vi "Read Transmission Spectrum.vi"(0 "VISA IN":refnum<visa-resource-name>="COM1" caption="serial number", 5 "error in (no error)":errorcluster caption="错误输入（无错误）") -> (14 "VISA OUT":refnum<visa-resource-name>, 15 "DATA":u8[](array[numeric]) format="%02x", 19 "error out":errorcluster caption="错误输出")   [LabVIEW 2013]
uses:
  <vilib>/Utility/file.llb/Write To Spreadsheet File (I64).vi
panel:
  out "Numeric":i32
  out "File path":path
  in  "Times":i32=10
  in  "STOP":bool
  out "XY Graph":cluster{i32[], u32[]}(graph)
  out "read buffer":string
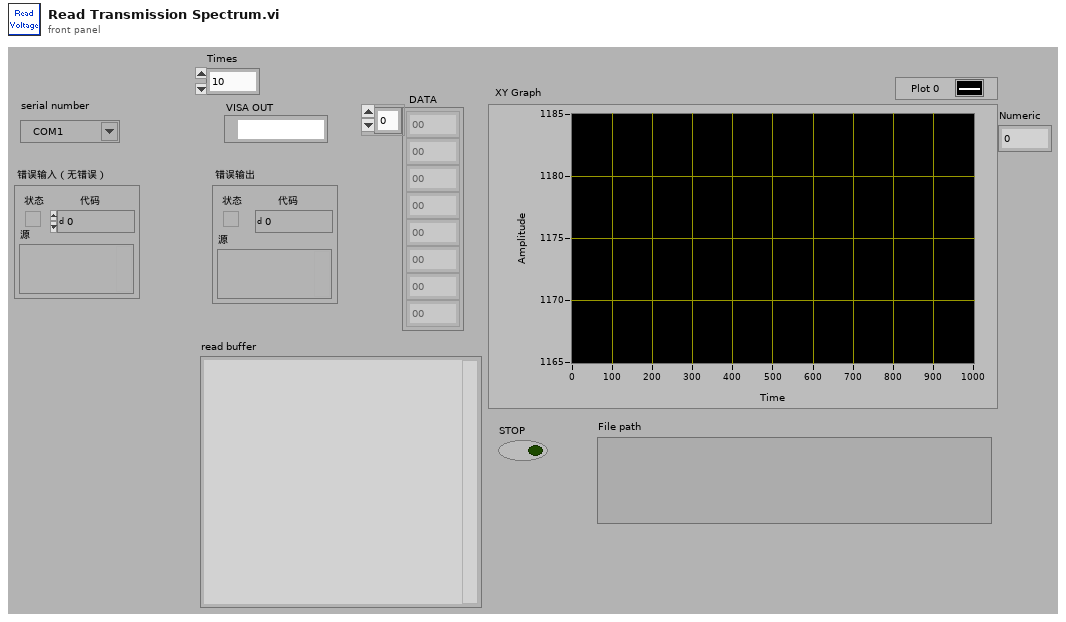
[diagram p1: front panel]
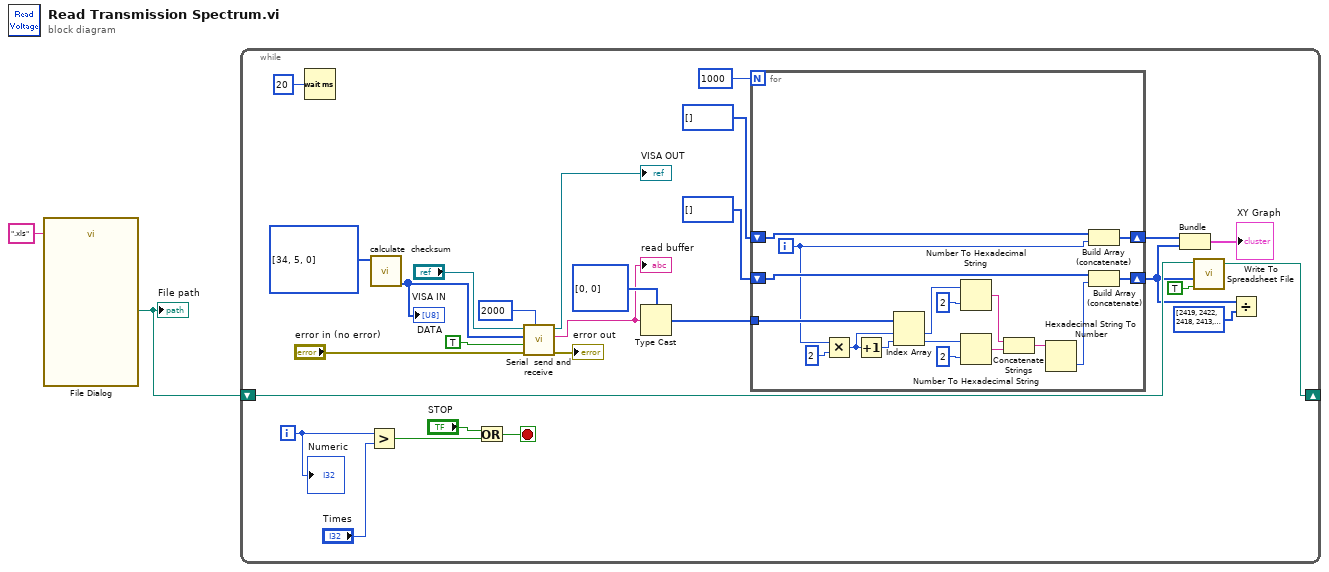
[diagram p0: block diagram]
diagram:
  n1 = call "File Dialog"("default name"=".xls") -> ("selected path"=w1:path)  [unwired: 11 in, 3 out]
  "File path" <- w1
  n2 = while {
    shift-right: [w6] -> _
    shift-left: w1 -> [w5]
    i -> [w10]
    stop <- w13 stop-if-true
    n3 = Wait (ms)(milliseconds to wait=u32 20) -> ()  [unwired: 1 out]
    n4 = Greater?(x=w10, y="Times") -> (0:w11:bool)
    n5 = call "calculate  checksum.vi"("front command"=u8[] [34, 5, 0]) -> ("DATA"=w29:u8[])  [unwired: 9 in, 1 out]
    "DATA" <- w29
    n6 = Or(x="STOP", y=w11) -> (x .or. y?=w13:bool)
    n7 = call "Serial  send and receive.vi"("读取字节总数"=u32 2000, "error in (no error)"="error in (no error)", "读取"=TRUE, "command"=w29, "VISA IN"="VISA IN") -> ("error out"=→"error out":errorcluster, "read buffer"=w14:string, "VISA OUT"=→"VISA OUT":refnum<visa-resource-name>)  [unwired: 2 in, 2 out]
    "read buffer" <- w14
    n8 = Type Cast(type=u8[] [0, 0], x=w14) -> (*(type *) &x=w20:u8[])
    n9 = for {
      N: 1000 -> [_]
      tunnel: w20 -> [w44]
      shift-right: [w35] -> w3
      shift-left: u32[] [] -> [w33]
      shift-right: [w31] -> w16
      shift-left: i32[] [] -> [w30]
      i -> [w32]
      n10 = Multiply(x=w32, y=i16 2 ("宽度(-)")) -> (x*y=w37:i32)
      n11 = Increment(x=w37) -> (x+1=w36:i32)
      n12 = Index Array(array=w44, index #1=w37, index #2=w36) -> (element #1=w46:u8, element #2=w43:u8)
      n13 = Number To Hexadecimal String(1:i16 2 ("宽度(-)"), 2:w46) -> (0:w45:string)
      n14 = Number To Hexadecimal String(1:i16 2 ("宽度(-)"), 2:w43) -> (0:w42:string)
      n15 = Concatenate Strings(w45, w42) -> (w39:string)
      n16 = Hexadecimal String To Number(string=w39) -> (number=w34:u32)  [unwired: 2 in, 1 out]
      n17 = Build Array (concatenate)(w30, w32) -> (w31:i32[])
      n18 = Build Array (concatenate)(w33, w34) -> (w35:u32[])
    }
    n19 = Bundle(w16, w3) -> (→"XY Graph":cluster{i32[], u32[]})  [unwired: 1 in]
    n20 = call-poly <vilib>:"Write To Spreadsheet File.vi"("append to file? (new file:F)"=TRUE, "1D data"=w3, "file path (dialog if empty)"=w5) -> ("new file path (Not A Path if cancelled)"=w6:path)  [unwired: 5 in]
    n21 = Divide(x=w3, y=u32[] [2419, 2422, 2418, 2413, 2407, 2401, 2394, 2390, 2384, 2380, 2372, 2366, 2351, 2347, 2343, 2338, 2334, 2327, 2321, 2317, 2316, 2311, 2305, 2301, 2294, 2289, 2285, 2281, 2276, 2272, 2268, 2266, 2260, 2255, 2253, 2249, 2246, 2243, 2237, 2233, 2231, 2226, 2222, 2218, 2216, 2213, 2207, 2206, 2203, 2198, 2196, 2192, 2191, 2187, 2185, 2182, 2176, 2177, 2175, 2175, 2170, 2166, 2161, 2160, 2155, 2152, 2149, 2149, 2146, 2142, 2141, 2139, 2137, 2135, 2134, 2131, 2127, 2125, 2124, 2122, 2120, 2118, 2116, 2114, 2110, 2110, 2109, 2108, 2105, 2102, 2104, 2098, 2101, 2097, 2094, 2093, 2098, 2093, 2093, 2092, 2087, 2085, 2083, 2082, 2082, 2081, 2080, 2079, 2077, 2076, 2074, 2073, 2073, 2071, 2060, 2069, 2069, 2068, 2069, 2066, 2065, 2065, 2065, 2063, 2063, 2061, 2058, 2060, 2058, 2057, 2056, 2056, 2059, 2056, 2059, 2056, 2058, 2057, 2052, 2052, 2052, 2053, 2052, 2052, 2052, 2051, 2051, 2049, 2051, 2050, 2048, 2050, 2051, 2049, 2049, 2049, 2047, 2048, 2048, 2048, 2048, 2047, 2047, 2048, 2047, 2047, 2049, 2047, 2047, 2048, 2046, 2048, 2048, 2049, 2050, 2050, 2050, 2046, 2047, 2047, 2045, 2048, 2035, 2047, 2044, 2048, 2048, 2049, 2048, 2048, 2049, 2048, 2048, 2048, 2048, 2049, 2050, 2049, 2049, 2048, 2048, 2049, 2049, 2048, 2052, 2050, 2050, 2049, 2049, 2051, 2052, 2056, 2055, 2056, 2056, 2053, 2054, 2053, 2055, 2054, 2054, 2055, 2055, 2056, 2052, 2057, 2056, 2056, 2059, 2058, 2057, 2057, 2060, 2058, 2059, 2060, 2060, 2060, 2061, 2062, 2063, 2063, 2064, 2065, 2064, 2066, 2064, 2066, 2066, 2069, 2069, 2072, 2070, 2069, 2069, 2069, 2069, 2070, 2071, 2072, 2072, 2071, 2073, 2072, 2073, 2075, 2076, 2077, 2076, 2077, 2078, 2077, 2078, 2078, 2078, 2081, 2078, 2079, 2081, 2083, 2083, 2082, 2085, 2084, 2085, 2085, 2085, 2088, 2088, 2088, 2092, 2087, 2089, 2089, 2089, 2090, 2091, 2093, 2092, 2093, 2093, 2096, 2095, 2098, 2095, 2097, 2098, 2098, 2098, 2100, 2098, 2100, 2102, 2102, 2102, 2102, 2104, 2103, 2104, 2104, 2107, 2107, 2107, 2108, 2110, 2113, 2113, 2114, 2114, 2112, 2110, 2115, 2113, 2114, 2116, 2114, 2117, 2117, 2118, 2118, 2118, 2118, 2120, 2119, 2122, 2123, 2122, 2123, 2124, 2127, 2126, 2126, 2127, 2128, 2129, 2128, 2131, 2131, 2132, 2131, 2133, 2133, 2134, 2134, 2138, 2138, 2138, 2140, 2138, 2139, 2139, 2140, 2140, 2142, 2141, 2142, 2142, 2143, 2144, 2143, 2144, 2145, 2148, 2146, 2148, 2149, 2148, 2150, 2150, 2139, 2149, 2150, 2153, 2154, 2153, 2153, 2156, 2154, 2157, 2158, 2159, 2161, 2163, 2163, 2163, 2164, 2163, 2161, 2164, 2164, 2164, 2166, 2168, 2167, 2168, 2167, 2168, 2169, 2170, 2171, 2170, 2173, 2177, 2172, 2172, 2175, 2175, 2178, 2177, 2179, 2177, 2179, 2179, 2181, 2184, 2182, 2183, 2184, 2185, 2185, 2189, 2189, 2189, 2189, 2189, 2188, 2190, 2189, 2190, 2192, 2192, 2192, 2192, 2195, 2196, 2194, 2195, 2196, 2197, 2200, 2198, 2199, 2201, 2201, 2200, 2201, 2203, 2204, 2203, 2206, 2204, 2207, 2210, 2208, 2208, 2208, 2210, 2210, 2214, 2214, 2216, 2214, 2214, 2214, 2205, 2216, 2218, 2218, 2218, 2220, 2219, 2220, 2221, 2222, 2222, 2222, 2224, 2225, 2226, 2226, 2225, 2228, 2227, 2228, 2228, 2229, 2230, 2230, 2231, 2232, 2235, 2235, 2235, 2235, 2235, 2234, 2236, 2240, 2240, 2242, 2243, 2241, 2241, 2242, 2241, 2243, 2242, 2243, 2244, 2246, 2244, 2247, 2247, 2246, 2248, 2248, 2251, 2249, 2251, 2252, 2252, 2251, 2252, 2253, 2255, 2255, 2256, 2258, 2255, 2259, 2260, 2258, 2260, 2259, 2260, 2263, 2263, 2263, 2263, 2263, 2264, 2265, 2267, 2269, 2256, 2269, 2269, 2270, 2270, 2270, 2272, 2272, 2275, 2273, 2276, 2275, 2275, 2276, 2276, 2277, 2278, 2276, 2279, 2280, 2278, 2282, 2282, 2283, 2282, 2285, 2285, 2285, 2286, 2289, 2289, 2289, 2290, 2277, 2290, 2289, 2290, 2290, 2293, 2290, 2293, 2292, 2293, 2294, 2296, 2295, 2295, 2297, 2297, 2297, 2297, 2299, 2300, 2301, 2301, 2302, 2304, 2301, 2302, 2303, 2305, 2305, 2304, 2304, 2305, 2307, 2304, 2309, 2308, 2311, 2309, 2309, 2309, 2311, 2314, 2312, 2313, 2314, 2314, 2312, 2314, 2314, 2315, 2316, 2318, 2318, 2317, 2319, 2318, 2318, 2321, 2321, 2322, 2322, 2322, 2322, 2325, 2323, 2325, 2326, 2325, 2323, 2324, 2325, 2328, 2329, 2330, 2330, 2334, 2334, 2330, 2331, 2331, 2330, 2332, 2332, 2334, 2333, 2334, 2334, 2333, 2334, 2337, 2338, 2339, 2336, 2338, 2339, 2339, 2339, 2339, 2340, 2342, 2344, 2343, 2343, 2345, 2346, 2346, 2347, 2347, 2348, 2347, 2349, 2348, 2351, 2353, 2350, 2351, 2351, 2349, 2352, 2352, 2354, 2352, 2353, 2352, 2355, 2356, 2357, 2357, 2359, 2355, 2359, 2360, 2359, 2361, 2360, 2361, 2360, 2362, 2362, 2363, 2365, 2363, 2364, 2365, 2365, 2368, 2368, 2366, 2365, 2371, 2371, 2371, 2372, 2371, 2370, 2371, 2372, 2372, 2372, 2372, 2375, 2372, 2373, 2374, 2377, 2374, 2375, 2376, 2376, 2376, 2377, 2378, 2378, 2378, 2378, 2380, 2380, 2380, 2381, 2381, 2381, 2383, 2384, 2385, 2384, 2385, 2383, 2387, 2385, 2385, 2385, 2385, 2386, 2388, 2388, 2388, 2388, 2389, 2389, 2388, 2388, 2390, 2389, 2394, 2391, 2392, 2393, 2393, 2394, 2393, 2394, 2393, 2395, 2396, 2397, 2396, 2396, 2397, 2397, 2399, 2399, 2398, 2399, 2401, 2398, 2405, 2405, 2403, 2405, 2402, 2401, 2400, 2404, 2403, 2403, 2404, 2404, 2404, 2405, 2404, 2405, 2403, 2404, 2407, 2399, 2406, 2406, 2408, 2409, 2407, 2409, 2409, 2409, 2409, 2410, 2408, 2409, 2409, 2410, 2411, 2413, 2413, 2416, 2413, 2416, 2418, 2418, 2418, 2414, 2417, 2415, 2416, 2416, 2417, 2418, 2418, 2417, 2417, 2418, 2418, 2418, 2419, 2418, 2419, 2420, 2421, 2420, 2419, 2421, 2422, 2420, 2422, 2421, 2420, 2422, 2423, 2422, 2424, 2421, 2424, 2422, 2422, 2424, 2424, 2425, 2424, 2422, 2424, 2423, 2425, 2425, 2423, 2424, 2423, 2424, 2425, 2423, 2422, 2424, 2422, 2422, 2420, 2422, 2422, 2422, 2422, 2422, 2423, 2423, 2421, 2422, 2422, 2421, 2424, 2422, 2424, 2422, 2421, 2424, 2423, 2424, 2424, 2425, 2424, 2422, 2424, 2424, 2421, 2422, 2422, 2422, 2422, 2420, 2420, 2421, 2420, 2422, 2421, 2421, 2419, 2420, 2419, 2420, 2420, 2419, 2421, 2420, 2421, 2418, 2418, 2420, 2420, 2420, 2421, 2420, 2420, 2420, 2418, 2418, 2418, 2421, 2421, 2419, 2418, 2418, 2418, 2416, 2416, 2417, 2418, 2418, 2415, 2415, 2414, 2414, 2415, 2414, 2414, 2415, 2414, 2413, 2412, 2416]) -> ()  [unwired: 1 out]
    "Numeric" <- w10
  }
